vi "Discrete Zero-Pole (DBL).vi"(2 "initialize":bool, 3 "gain-zeros-poles":T1 {"poles" format="%.2f"; "zeros" format="%.2f"; "gain" format="%.2f"}, 5 "input point":dbl format="%.2f") -> (1 "output point":dbl format="%.2f")   [LabVIEW 2020, in "NI_AdvCtrl_discrete linear.lvlib"]
doc: "LabVIEW no longer supports this VI. You can obtain similar functionality by installing the LabVIEW Simulation Module.\n\nCalculates the new output point, where the discrete transfer function and the input point are given. The discrete transfer function is described in gain-zeros-poles notation."
uses:
  <vilib>/addons/control/advanced/NI_AdvCtrl_discrete linear.lvlib
  <vilib>/addons/control/advanced/NI_AdvCtrl_continuous linear.lvlib
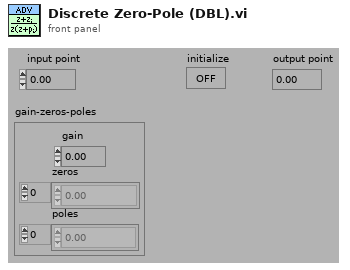
[diagram p1: front panel]
types:
  T1 = cluster{"gain":dbl, "zeros":cdb[], "poles":cdb[]}
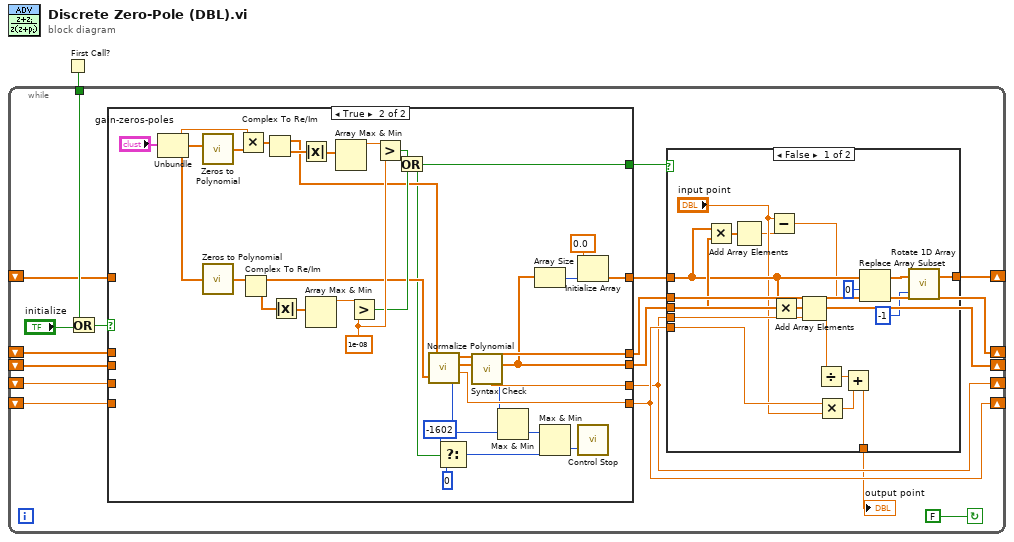
[diagram p0: block diagram]
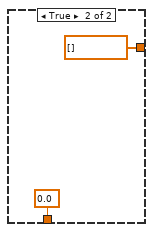
[diagram p2: hidden frame]
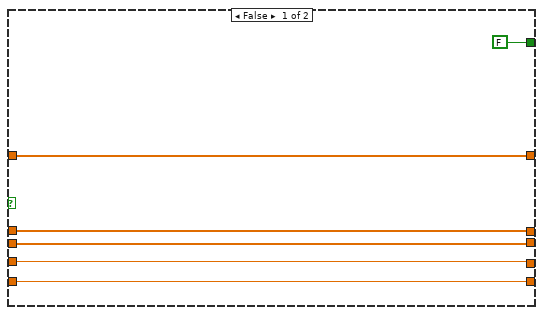
[diagram p3: hidden frame]
diagram:
  n1 = First Call?() -> (First Call?: T/F=w1:bool)
  n2 = while {
    shift-left: _ -> [w7]
    shift-right: [w8] -> _
    tunnel: w1 -> [w10]
    shift-left: _ -> [w15]
    shift-right: [w14] -> _
    shift-left: _ -> [w16]
    shift-right: [w13] -> _
    shift-left: _ -> [w17]
    shift-right: [w5] -> _
    shift-left: _ -> [w18]
    shift-right: [w6] -> _
    stop <- FALSE continue-if-true
    n3 = Or(x=w10, y="initialize") -> (x .or. y?=w9:bool)
    n4 = case shown="True" w9 {
      tunnel: [w41 w77] -> w14
      tunnel: [w42 w76] -> w13
      tunnel: [w44 w75] -> w6
      tunnel: [w43 w72] -> w5
      tunnel: w18 -> [w44 _]
      tunnel: w17 -> [w43 _]
      tunnel: w16 -> [w42 _]
      tunnel: w15 -> [w41 _]
      tunnel: [w40 w71] -> w4
      tunnel: w7 -> [w40 _]
      tunnel: [FALSE w50] -> w2
      frame False {
      }
      frame True {
        w65 = 1e-08
        n5 = Unbundle("gain-zeros-poles") -> ("gain"=w53:dbl, "zeros"=w56:cdb[], "poles"=w55:cdb[])
        n6 = call <vilib>:"Zeros to Polynomial.vi"("Zeros"=w56) -> ("Polynomial"=w54:cdb[])
        n7 = call <vilib>:"Zeros to Polynomial.vi"("Zeros"=w55) -> ("Polynomial"=w69:cdb[])
        n8 = Multiply(x=w53, y=w54) -> (x*y=w70:cdb[])
        n9 = Complex To Re/Im(x + iy=w69) -> (x=w58:dbl[], y=w67:dbl[])
        n10 = Complex To Re/Im(x + iy=w70) -> (x=w59:dbl[], y=w61:dbl[])
        n11 = Absolute Value(x=w67) -> (abs(x)=w68:dbl[])
        n12 = Absolute Value(x=w61) -> (abs(x)=w62:dbl[])
        n13 = Array Max & Min(array=w68) -> (max value=w66:dbl)  [unwired: 3 out]
        n14 = Array Max & Min(array=w62) -> (max value=w60:dbl)  [unwired: 3 out]
        n15 = Greater?(x=w66, y=w65) -> (0:w64:bool)
        n16 = Greater?(x=w60, y=w65) -> (0:w63:bool)
        n17 = Or(x=w63, y=w64) -> (x .or. y?=w50:bool)
        n18 = call <vilib>:"Normalize Polynomial.vi"("Numerator"=w59, "Denominator"=w58) -> ("Numerator new"=w78:dbl[], "Denominator new"=w79:dbl[], "additive constant"=w77:dbl, "error"=w51:i32)
        n19 = Select(t=-1602, s=w50, f=0) -> (s? t:f=w46:i32)
        n20 = call <vilib>:"Syntax Check.vi"("Denominator"=w79, "Numerator"=w78) -> ("error"=w52:i32, "gain"=w76:dbl, "Denominator new"=w72:dbl[], "Numerator new"=w75:dbl[])  [unwired: 1 out]
        n21 = Max & Min(x=w52, y=w51) -> (min(x,y)=w47:i32)  [unwired: 1 out]
        n22 = Array Size(array=w72) -> (size(s)=w73:i32)
        n23 = Max & Min(x=w47, y=w46) -> (min(x,y)=w45:i32)  [unwired: 1 out]
        n24 = Initialize Array(0.0, w73) -> (w71:dbl[])
        n25 = call <vilib>:"Control Stop.vi"("error"=w45) -> ()  [unwired: 2 out]
      }
    }
    n26 = case shown="False" w2 {
      tunnel: w14 -> [w36 _]
      tunnel: w13 -> [w35 _]
      tunnel: [w21 dbl[] []] -> w8
      tunnel: w6 -> [w34 _]
      tunnel: w5 -> [w33 _]
      tunnel: w4 -> [w32 _]
      tunnel: [w22 0.0] -> w3
      frame False {
        n27 = Multiply(x=w32, y=w33) -> (x*y=w24:dbl[])
        n28 = Add Array Elements(numeric array=w24) -> (sum=w23:dbl)
        n29 = Subtract(x="input point", y=w23) -> (x-y=w29:dbl)
        n30 = Multiply(x=w32, y=w34) -> (x*y=w27:dbl[])
        n31 = Add Array Elements(numeric array=w27) -> (sum=w26:dbl)
        n32 = Divide(x=w26, y=w35) -> (x/y=w30:dbl)
        n33 = Multiply(x=w36, y="input point") -> (x*y=w31:dbl)
        n34 = Add(x=w30, y=w31) -> (x+y=w22:dbl)
        n35 = Replace Array Subset(array=w32, new element=w29, index=0 ("Index")) -> (w20:dbl[])
        n36 = call <vilib>:"Rotate 1D Array.vi"("n"=-1, "array"=w20) -> ("array (last n elements first)"=w21:dbl[])  [unwired: 1 out]
      }
      frame True {
      }
    }
    "output point" <- w3
  }
